vi "oa_No Pulse or Max Order Change Reset.vi"(8 "max order (auto)":i32, 10 "speed profile in":T1 {"speed [RPM]" format="%.2f"; "time [s]" format="%.2f"}, 11 "reset? (T)":bool=TRUE) -> (2 "speed profile out":T1 {"speed [RPM]" format="%.2f"; "time [s]" format="%.2f"}, 3 "reset out":bool)   [LabVIEW 2017, in "SoundVib_Resampling.lvlib"]
uses:
  <vilib>/addons/Sound and Vibration/Order Analysis/Resample Order Tracking/SoundVib_Resampling.lvlib
  <vilib>/addons/Sound and Vibration/Order Analysis/Tach Process/SubVIs/speed profile.ctl
  <vilib>/addons/Sound and Vibration/Order Analysis/Tach Process/SoundVib_TachProcess.lvlib
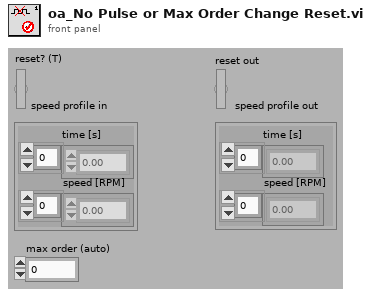
[diagram p1: front panel]
types:
  T1 = typedef "SoundVib_TachProcess.lvlib/speed profile.ctl" = cluster{"time [s]":dbl[], "speed [RPM]":dbl[]}
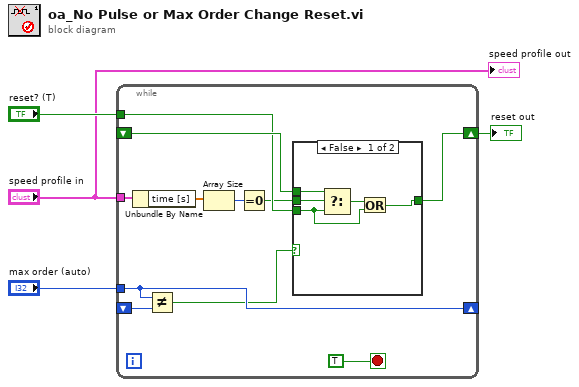
[diagram p0: block diagram]
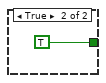
[diagram p2: hidden frame]
diagram:
  n1 = while {
    shift-right: [w11] -> _
    shift-left: _ -> [w10]
    tunnel: "max order (auto)" -> [w11]
    tunnel: "speed profile in" -> [w14]
    tunnel: "reset? (T)" -> [w7]
    shift-right: [w5] -> w1
    shift-left: _ -> [w8]
    stop <- TRUE stop-if-true
    n2 = Unbundle By Name(w14) -> ("time [s]"=w13:dbl[])
    n3 = Not Equal?(x=w11, y=w10) -> (x != y?=w9:bool)
    n4 = Array Size(array=w13) -> (size(s)=w12:i32)
    n5 = Equal To 0?(x=w12) -> (x = 0?=w6:bool)
    n6 = case shown="False" w9 {
      tunnel: w8 -> [w19 _]
      tunnel: w7 -> [w17 _]
      tunnel: w6 -> [w20 _]
      tunnel: [w16 TRUE] -> w5
      frame False {
        n7 = Select(t=w19, s=w20, f=w17) -> (s? t:f=w18:bool)
        n8 = Or(x=w18, y=w17) -> (x .or. y?=w16:bool)
      }
      frame True {
      }
    }
  }
  "reset out" <- w1
  "speed profile out" <- "speed profile in"
